vi "crc-16 (SubVI).vi"(0 "String":string) -> (1 "CRC =":u16 format="%x", 2 "hex integer string":string)   [LabVIEW 2012]
panel:
  # "Polynom X16+X12+X5+1"
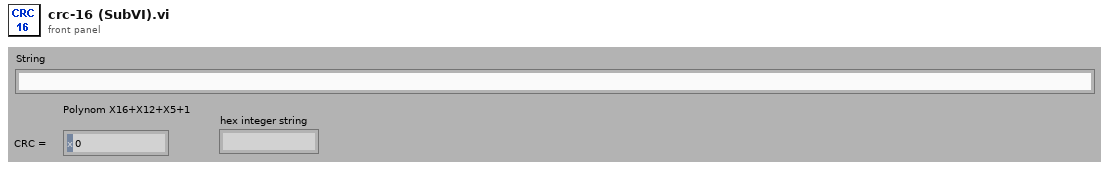
[diagram p1: front panel]
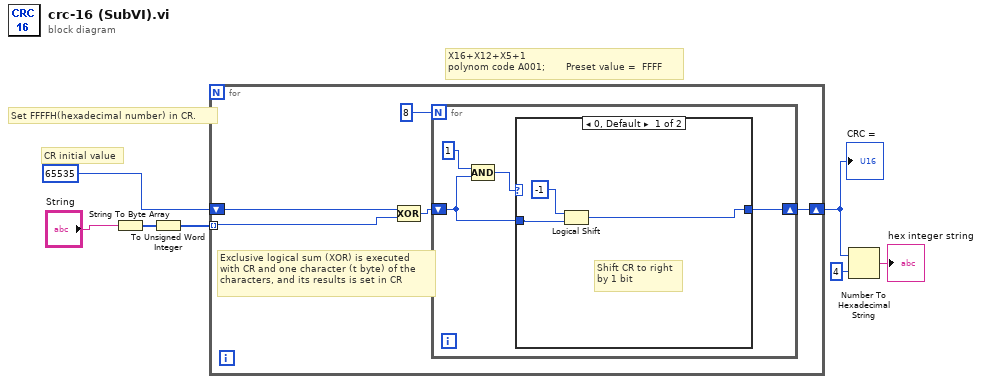
[diagram p0: block diagram]
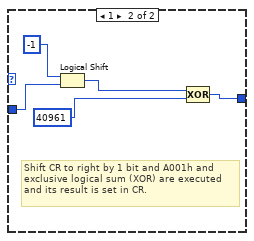
[diagram p2: hidden frame]
diagram:
  # "Set FFFFH(hexadecimal number) in CR."
  # "CR initial value"
  # "X16+X12+X5+1\npolynom code A001;       Preset value =  FFFF"
  n1 = String To Byte Array(string="String") -> (unsigned byte array=w6:u8[])
  n2 = To Unsigned Word Integer(number=w6) -> (unsigned 16bit integer=w5:u16[])
  n3 = for {
    shift-right: [w9] -> w3
    shift-left: u16 65535 -> [w10]
    tunnel: w5 -> [w8] mode=indexing
    # "Exclusive logical sum (XOR) is executed\nwith CR and one character (t byte) of the\ncharacters, and its results is set in CR"
    n4 = Compound Arithmetic op=XOR(w10, w8) -> (w11:u32)
    n5 = for {
      N: 8 -> [_]
      shift-right: [w15] -> w9
      shift-left: w11 -> [w14]
      n6 = Compound Arithmetic op=AND(u16 1, w14) -> (w13:u32)
      n7 = case shown="0, Default" w13 {
        tunnel: [w18 w23] -> w15
        tunnel: w14 -> [w17 w20]
        frame 0, Default {
          # "Shift CR to right\nby 1 bit"
          n8 = Logical Shift(y=i16 -1, x=w17) -> (x << y=w18:u32)
        }
        frame 1 {
          # "Shift CR to right by 1 bit and A001h and\nexclusive logical sum (XOR) are executed\nand its result is set in CR."
          n9 = Logical Shift(y=i16 -1, x=w20) -> (x << y=w22:u32)
          n10 = Compound Arithmetic op=XOR(w22, u32 40961) -> (w23:u32)
        }
      }
    }
  }
  "CRC =" <- w3
  n11 = Number To Hexadecimal String(1:i16 4 ("width (-)"), 2:w3) -> (0:→"hex integer string":string)
